vi "read_str_from_bl.vi"(2 "[ESC]":bool, 3 "RESET MODULE":bool, 5 "CTS":bool) -> (1 "INC STRING":string)   [LabVIEW 2019]
uses:
  <vilib>/myRIO/Instrument Drivers/Utilities/Utilities.lvlib
  <vilib>/Instr/_visa.llb/VISA Configure Serial Port (Instr).vi
panel:
  out "READ INC DATA MODE":bool
  out "incoming\ncharacter":string
  out "RTS":bool
  out "STATUS":bool
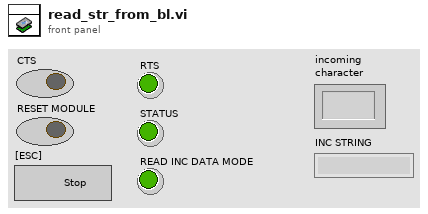
[diagram p1: front panel]
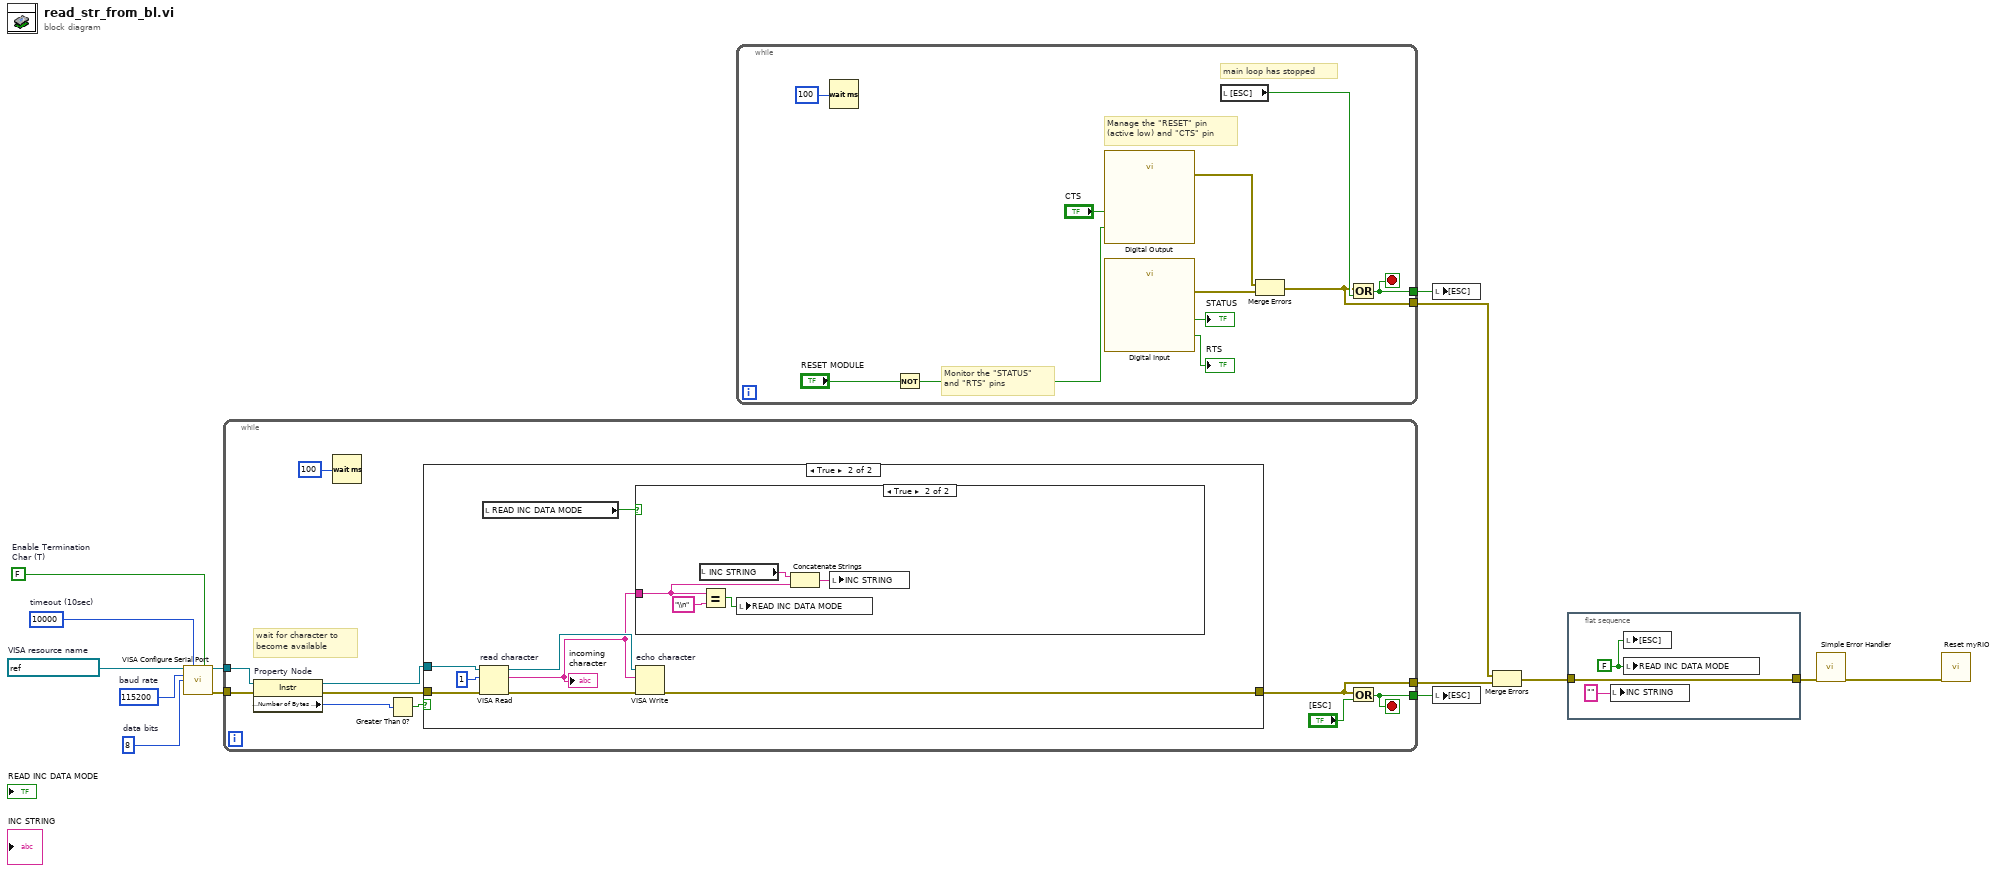
[diagram p0: block diagram]
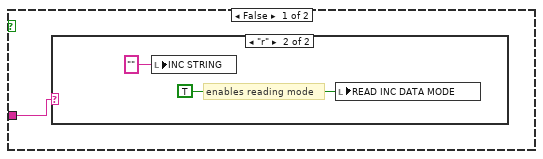
[diagram p3: hidden frame]
diagram:
  w1 = u32 10000  # timeout (10sec)
  w4 = FALSE  # Enable Termination Char (T)
  w10 = u16 8  # data bits
  w11 = u32 115200  # baud rate
  w13 = refnum<visa-resource-name> "ASRL2::INSTR"  # VISA resource name
  n1 = call-poly "VISA Configure Serial Port"("VISA resource name"=w13, "timeout (10sec)"=w1, "Enable Termination\nChar (T)"=w4, "baud rate (9600)"=w11, "data bits (8)"=w10) -> ("VISA resource name out"=w12:refnum<visa-resource-name>, "error out"=w7:errorcluster)  [unwired: 9 in]
  n2 = while {
    tunnel: [w22] -> w9
    tunnel: w12 -> [w20]
    tunnel: w7 -> [w19]
    tunnel: [w21] -> w6
    stop <- w21 stop-if-true
    # "wait for character to\nbecome available"
    n3 = property on="Property Node" class="Instr"(reference=w20, error in=w19) -> (reference out=w15:refnum<visa-resource-name>, error out=w18:errorcluster, "Serial Settings:Number of Bytes at Serial Port"=w17:u32)
    n4 = Wait (ms)(milliseconds to wait=u32 100) -> ()  [unwired: 1 out]
    n5 = Greater Than 0?(x=w17) -> (x > 0?=w16:bool)
    n6 = case shown="True" w16 {
      tunnel: [w25 w28] -> w22
      tunnel: w18 -> [w25 w32]
      tunnel: w15 -> [_ w31]
      frame False {
      }
      frame True {
        n7 = VISA Read "read character"(VISA resource name=w31, byte count=u32 1, error in (no error)=w32) -> (VISA resource name out=w29:refnum<visa-resource-name>, read buffer=w26:string, error out=w30:errorcluster)  [unwired: 1 out]
        "incoming\ncharacter" <- w26
        n8 = local read "READ INC DATA MODE"() -> (w27:bool)
        n9 = case shown="True" w27 {
          tunnel: w26 -> [w34 w37]
          frame False {
            n10 = case shown="\"r\"" w34 {
              frame Default {
              }
              frame "r" {
                # "enables reading mode"
                n11 = local write "INC STRING"("" ("INC STRING")) -> ()
                n12 = local write "READ INC DATA MODE"(TRUE) -> ()
              }
            }
          }
          frame True {
            n13 = local read "INC STRING"() -> (w39:string)
            n14 = Equal?(x=w37, y="\\n") -> (x = y?=w40:bool)
            n15 = local write "READ INC DATA MODE"(w40) -> ()
            n16 = Concatenate Strings(w39, w37) -> (w38:string)
            n17 = local write "INC STRING"(w38) -> ()
          }
        }
        n18 = VISA Write "echo character"(VISA resource name=w29, write buffer=w26, error in (no error)=w30) -> (error out=w28:errorcluster)  [unwired: 2 out]
      }
    }
    n19 = Or(x=w22, y="[ESC]") -> (x .or. y?=w21:bool)
  }
  n20 = while {
    tunnel: [w47] -> w8
    tunnel: [w49] -> w5
    stop <- w49 stop-if-true
    # "Manage the \"RESET\" pin\n(active low) and \"CTS\" pin"
    # "main loop has stopped"
    # "Monitor the \"STATUS\"\nand \"RTS\" pins"
    n21 = Wait (ms)(milliseconds to wait=u32 100) -> ()  [unwired: 1 out]
    n22 = Not(x="RESET MODULE") -> (.not. x?=w43:bool)
    n23 = call "Digital Output"("B/DIO2 (Pin 15)"="CTS", "B/DIO3 (Pin 17)"=w43) -> ("error out"=w48:errorcluster)  [unwired: 25 in]
    n24 = call "Digital Input"() -> ("B/DIO0 (Pin 11)"=→"STATUS":bool, "B/DIO1 (Pin 13)"=→"RTS":bool, "error out"=w44:errorcluster)  [unwired: 25 in]
    n25 = local read "[ESC]"() -> (w50:bool)
    n26 = Merge Errors "Merge Errors"(w48, w44) -> (w47:errorcluster)
    n27 = Or(x=w47, y=w50) -> (x .or. y?=w49:bool)
  }
  n28 = local write "[ESC]"(w5) -> ()
  n29 = local write "[ESC]"(w6) -> ()
  n30 = Merge Errors "Merge Errors"(w8, w9) -> (w3:errorcluster)
  n31 = flat-sequence {
    tunnel: w3 -> [w55]
    tunnel: [w55] -> w2
    frame #0 {
      w54 = FALSE ("[ESC]")
      n32 = local write "INC STRING"("" ("INC STRING")) -> ()
      n33 = local write "[ESC]"(w54) -> ()
      n34 = local write "READ INC DATA MODE"(w54) -> ()
    }
  }
  n35 = call <vilib>:"Simple Error Handler.vi"("error in (no error)"=w2) -> ("error out"=w14:errorcluster)  [unwired: 4 in, 4 out]
  n36 = call <vilib>:"Reset myRIO.vi"("error in (no error)"=w14) -> ()  [unwired: 10 in, 1 out]
